vi "Create Plots - 2D, 3D (SubVI).vi"(0 "Array in":u32[](array[numeric]), 1 "milliseconds to wait":u32, 5 "X array in":dbl[](array[numeric]), 7 "Y array in":dbl[](array[numeric]), 9 "NavData Out":T1, 12 "Numeric 2":dbl, 13 "Numeric":dbl) -> (3 "3D Graph":refnum<class "Base Datatype.lvclass">[](array[class]), 4 "XY Graph":cluster{"Y":dbl[], "Y":dbl[]}[](array[cluster]), 6 "Array out":u32[](array[numeric]), 8 "X array out":dbl[](array[numeric]), 10 "Y array out":dbl[](array[numeric]), 15 "error out":errorcluster)   [LabVIEW 2014]
uses:
  <vilib>/Native 3D Graph/classes/Base Datatype.lvclass
  <vilib>/LVH/AR Drone Toolkit/Decode NavData/Typedefs/NavData Demo.ctl
  <vilib>/LVH/AR Drone Toolkit/AR Drone.lvlib
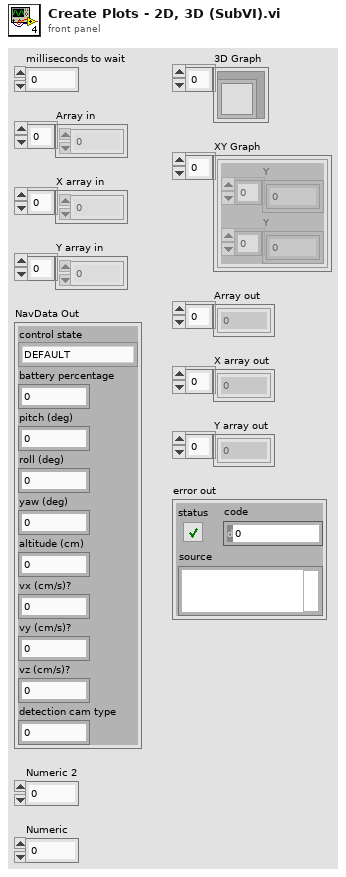
[diagram p1: front panel]
types:
  T1 = typedef "AR Drone.lvlib/NavData Demo.ctl" = cluster{"control state":enum32{"DEFAULT", "INIT", "LANDING", "FLYING", "HOVERING", "TEST", "TRANS_TAKEOFF", "TRANS_GOTOFIX", "TRANS_LANDING"}, "battery percentage":u32, "pitch (deg)":sgl, "roll (deg)":sgl, "yaw (deg)":sgl, "altitude (cm)":u32, "vx (cm/s)?":sgl, "vy (cm/s)?":sgl, "vz (cm/s)?":sgl, "detection cam type":u32}
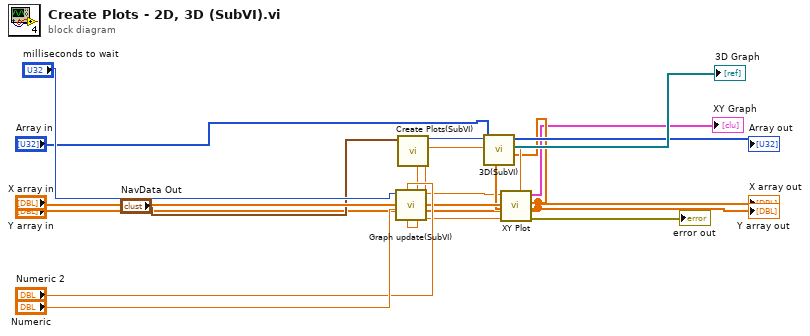
[diagram p0: block diagram]
diagram:
  n1 = call "Create Plots(SubVI).vi"("NavData Out"="NavData Out") -> ("Numeric 2"=w4:sgl, "yaw (deg)"=w10:sgl, "altitude (cm)"=w12:u32, "Numeric"=w5:sgl)  [unwired: 7 in]
  n2 = call "Graph update(SubVI).vi"("vy (cm/s)?"=w5, "Numeric 4"="Numeric 2", "Numeric in"="Numeric", "vx (cm/s)?"=w4, "milliseconds to wait"="milliseconds to wait") -> ("Numeric out"=w2:dbl, "Numeric 3"=w1:dbl)  [unwired: 5 in]
  n3 = call "XY Plot.vi"("X"=w1, "X array"="X array in", "Y array"="Y array in", "Y"=w2, "Angle"=w10) -> ("XY Graph"=→"XY Graph":cluster{"Y":dbl[], "Y":dbl[]}[], "X array"=w7:dbl[], "Y array"=w8:dbl[], "error out"=→"error out":errorcluster)  [unwired: 1 out]
  "Y array out" <- w8
  "X array out" <- w7
  n4 = call "3D(SubVI).vi"("Y array"=w8, "X array"=w7, "Array in"="Array in", "altitude (cm)"=w12) -> ("3D Graph"=→"3D Graph":refnum<class "Base Datatype.lvclass">[], "Array out"=→"Array out":u32[])  [unwired: 6 in]
